vi "Init.vi"(7 "I2C #":T2=-1, 8 "error in (no error)":errorcluster, 9 "Range Mode":T1=enum."Single", 10 "Session In":refnum<class "Session.lvclass">) -> (0 "error out":errorcluster, 3 "Grove Ranging Sensor VL53L0X Out":refnum<class "Grove Range Sensor VL53L0X .lvclass">)   [LabVIEW 2020, in "CTI-Peripheral.lvlib" / "Grove Range Sensor VL53L0X .lvclass"]
uses:
  Grove Range Sensor VL53L0X .lvclass
  CTI/Session/Session.lvclass
  CTI/I2C Number.ctl
  Private/Range Mode.ctl
  CTI/I2C Address.ctl
  CTI/I2C Connection/I2C Connection.lvclass/I2C Connection.ctl
  Grove Range Sensor VL53L0X .lvclass/Grove Range Sensor VL53L0X .ctl
  CTI/I2C Connection/I2C Connection.lvclass
  CTI/CTI.lvlib
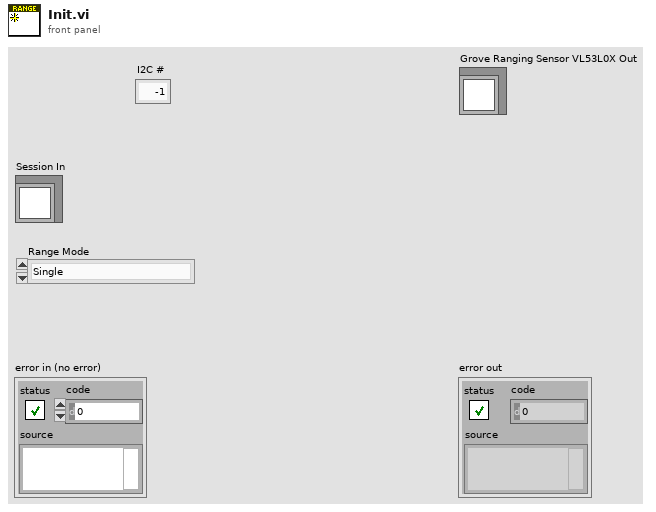
[diagram p1: front panel]
types:
  T1 = typedef "CTI-Peripheral.lvlib/Grove Range Sensor VL53L0X .lvclass/Range Mode.ctl" = enum16{"No Mode - Error", "Single", "Continuous", "High Speed", "High Accuracy", "Long Distance"}
  T2 = typedef "CTI.lvlib/I2C Number.ctl" = i8
  T3 = typedef "CTI.lvlib/I2C Address.ctl" = u8
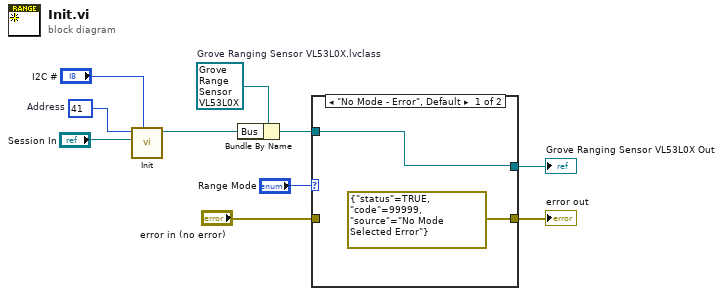
[diagram p0: block diagram]
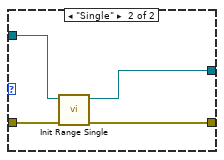
[diagram p2: hidden frame]
diagram:
  w6 = refnum<class "Grove Range Sensor VL53L0X .lvclass"> refnum  # Grove Ranging Sensor VL53L0X.lvclass
  w7 = T3 41  # Address
  n1 = call "Init.vi"("I2C #"="I2C #", "Session"="Session In", "Address"=w7) -> ("I2C Connection"=w10:refnum<class "I2C Connection.lvclass">)  [unwired: 7 in, 1 out]
  n2 = Bundle By Name(cluster=w6, "Bus"=w10) -> (w5:refnum<class "Grove Range Sensor VL53L0X .lvclass">)
  n3 = case shown="\"No Mode - Error\", Default" "Range Mode" {
    tunnel: w5 -> [w12 w16]
    tunnel: [w12 w15] -> w4
    tunnel: "error in (no error)" -> [_ w14]
    tunnel: [errorcluster {"status"=TRUE, "code"=99999, "source"="No Mode Selected Error"} ("error out") w13] -> w2
    frame "No Mode - Error", Default {
    }
    frame "Single" {
      n4 = call "Init Range Single.vi"("error in (no error)"=w14, "Grove Ranging Sensor VL53L0X in"=w16) -> ("error out"=w13:errorcluster, "Grove Ranging Sensor VL53L0X out"=w15:refnum<class "Grove Range Sensor VL53L0X .lvclass">)  [unwired: 8 in]
    }
  }
  "error out" <- w2
  "Grove Ranging Sensor VL53L0X Out" <- w4
